vi "S4GUI.vi"(7 "Tab ObsEng":enum32{"Obs", "CCD modes", "Eng"}(tab)) -> ()   [LabVIEW 2018] (continued)
            n3430 = call-dynamic "Read Channel.vi"("error in (no error)"=w7850, "Acquisition in"=w7851) -> ("error out"=w7852:errorcluster, "Channel.lvclass"=w7853:refnum<class "Channel.lvclass">, "Acquisition out"=w7864:refnum<class "Acquisition.lvclass">)  [unwired: 7 in]
            n3431 = call-dynamic "Read Interface.vi"("error in (no error)"=w7852, "Channel in"=w7853) -> ("error out"=w7874:errorcluster, "Interface.lvclass"=w7875:refnum<class "Interface.lvclass">, "Channel out"=w7873:refnum<class "Channel.lvclass">)  [unwired: 7 in]
            n3432 = call "Write Exposure Time.vi"("error in (no error)"=w7874, "Exposure Time"="Exptime ch1", "Interface in"=w7875) -> ("error out"=w7820:errorcluster, "Interface out"=w7821:refnum<class "Interface.lvclass">)  [unwired: 7 in]
            n3433 = case shown="Default" w7807 {
              tunnel: w7821 -> [w7902 w7907]
              tunnel: w7820 -> [w7901 w7906]
              tunnel: "Exptime ch1" -> [_ w7905]
              tunnel: [w7901 w7904] -> w7818
              tunnel: [w7902 w7903] -> w7817
              frame "ZERO" {
              }
              frame Default {
                n3434 = call-dynamic "Write prev ExpTime.vi"("error in (no error)"=w7906, "prev ExpTime"=w7905, "Interface in"=w7907) -> ("error out"=w7904:errorcluster, "Interface out"=w7903:refnum<class "Interface.lvclass">)  [unwired: 7 in]
              }
            }
            n3435 = call-dynamic "Write Suffix.vi"("error in (no error)"=w7818, "Suffix"=w7849, "Interface in"=w7817) -> ("error out"=w7872:errorcluster, "Interface out"=w7871:refnum<class "Interface.lvclass">)  [unwired: 7 in]
            n3436 = call-dynamic "Write ObsType.vi"("error in (no error)"=w7872, "ObsType"=w7847, "Interface in"=w7871) -> ("error out"=w7869:errorcluster, "Interface out"=w7870:refnum<class "Interface.lvclass">)  [unwired: 7 in]
            n3437 = call-dynamic "Write Object.vi"("error in (no error)"=w7869, "Object"=w7846, "Interface in"=w7870) -> ("error out"=w7868:errorcluster, "Interface out"=w7867:refnum<class "Interface.lvclass">)  [unwired: 7 in]
            n3438 = call-dynamic "Write Comments.vi"("error in (no error)"=w7868, "Comments"=w7848, "Interface in"=w7867) -> ("error out"=w7865:errorcluster, "Interface out"=w7866:refnum<class "Interface.lvclass">)  [unwired: 7 in]
            n3439 = call-dynamic "Write DS9.vi"("error in (no error)"=w7865, "DS9"="F", "Interface in"=w7866) -> ("error out"=w7843:errorcluster, "Interface out"=w7845:refnum<class "Interface.lvclass">)  [unwired: 7 in]
            n3440 = call-dynamic "Write Observer.vi"("error in (no error)"=w7843, "Observer"=w7841, "Interface in"=w7845) -> ("error out"=w7842:errorcluster, "Interface out"=w7844:refnum<class "Interface.lvclass">)  [unwired: 7 in]
            n3441 = call-dynamic "Write # Images.vi"("error in (no error)"=w7842, "# Images"="Exp ch1", "Interface in"=w7844) -> ("error out"=w7861:errorcluster, "Interface out"=w7863:refnum<class "Interface.lvclass">)  [unwired: 7 in]
            n3442 = call-dynamic "Write Interface.vi"("error in (no error)"=w7861, "Interface.lvclass"=w7863, "Channel in"=w7873) -> ("error out"=w7854:errorcluster, "Channel out"=w7855:refnum<class "Channel.lvclass">)  [unwired: 7 in]
            n3443 = property on="Exposure Time ch1" class="Slide (strict)"("Scale.Maximum"="Exptime ch1", "Scale.Minimum"=0.0 ("Scale.Range:Minimum")) -> ()  [unwired: 2 in, 2 out]
            n3444 = property on="Cycles Done ch1" class="Slide (strict)"("Scale.Maximum"=w7832, "Scale.Minimum"=0.0 ("Scale.Range:Minimum")) -> ()  [unwired: 2 in, 2 out]
            n3445 = property on="Exposures Done ch1" class="Slide (strict)"("Scale.Maximum"="Exp ch1", "Scale.Minimum"=0.0 ("Scale.Range:Minimum")) -> ()  [unwired: 2 in, 2 out]
            n3446 = call-dynamic "Write ciclos.vi"("error in (no error)"=w7854, "ciclos"=w7832, "Channel in"=w7855) -> ("error out"=w7839:errorcluster, "Channel out"=w7840:refnum<class "Channel.lvclass">)  [unwired: 7 in]
            n3447 = call-dynamic "Write sequencias.vi"("error in (no error)"=w7839, "sequencias"=w7822, "Channel in"=w7840) -> ("error out"=w7838:errorcluster, "Channel out"=w7837:refnum<class "Channel.lvclass">)  [unwired: 7 in]
            n3448 = call-dynamic "Write Channel.vi"("error in (no error)"=w7838, "Channel.lvclass"=w7837, "Acquisition in"=w7864) -> ("error out"=w7805:errorcluster, "Acquisition out"=w7806:refnum<class "Acquisition.lvclass">)  [unwired: 7 in]
            n3449 = call-dynamic "CalcCubeDuration.vi"("error in (no error)"=w7805, "Acquisition in"=w7806) -> ("error out"=w7803:errorcluster, "Acquisition out"=w7804:refnum<class "Acquisition.lvclass">)  [unwired: 8 in]
            n3450 = call-dynamic "Write sequencias.vi"("error in (no error)"=w7803, "sequencias"=w7822, "S4GUI in"=w7813) -> ("error out"=w7834:errorcluster, "S4GUI out"=w7833:refnum<class "S4GUI.lvclass">)  [unwired: 7 in]
            n3451 = call-dynamic "Write ciclos.vi"("error in (no error)"=w7834, "ciclos"=w7832, "S4ACS_GUI in"=w7833) -> ("error out"=w7835:errorcluster, "S4ACS_GUI out"=w7836:refnum<class "S4GUI.lvclass">)  [unwired: 7 in]
            n3452 = call-dynamic "Write TotalCiclos.vi"("error in (no error)"=w7835, "TotalCiclos"=w7832, "S4GUI in"=w7836) -> ("error out"=w7830:errorcluster, "S4GUI out"=w7831:refnum<class "S4GUI.lvclass">)  [unwired: 7 in]
          }
        }
        n3453 = call-dynamic "Write AcquisitionA.vi"("error in (no error)"=w7748, "Acquisition.lvclass"=w7763, "S4ACS_GUI in"=w7764) -> ("error out"=w7749:errorcluster, "S4ACS_GUI out"=w7750:refnum<class "S4GUI.lvclass">)  [unwired: 7 in]
      }
      event "Start ch2": Value Change {
        n3454 = event-data() -> ()  [unwired: 1 in, 6 out]
        n3455 = call "Read Instrument.lvclass.vi"("error in (no error)"=w7916, "S4ACS_GUI in"=w7917) -> ("error out"=w7918:errorcluster, "Instrument.lvclass"=w7919:refnum<class "Instrument.lvclass">, "S4ACS_GUI out"=w7915:refnum<class "S4GUI.lvclass">)  [unwired: 7 in]
        n3456 = call-dynamic "Read mode.vi"("error in (no error)"=w7918, "Instrument in"=w7919) -> ("error out"=w7914:errorcluster, "mode"=w7913:bool)  [unwired: 7 in, 1 out]
        n3457 = call "Read AcquisitionB.vi"("error in (no error)"=w7914, "S4ACS_GUI in"=w7915) -> ("error out"=w7933:errorcluster, "Acquisition.lvclass"=w7934:refnum<class "Acquisition.lvclass">, "S4ACS_GUI out"=w7936:refnum<class "S4GUI.lvclass">)  [unwired: 7 in]
        n3458 = call-dynamic "Read Acq_state.vi"("error in (no error)"=w7933, "Acquisition in"=w7934) -> ("error out"=w7930:errorcluster, "Acq_state"=w7932:u32, "Acquisition out"=w7929:refnum<class "Acquisition.lvclass">)  [unwired: 7 in]
        n3459 = Not Equal?(x=w7932, y=u32 400) -> (x != y?=w7935:bool)
        n3460 = case shown="True" w7935 {
          tunnel: w7936 -> [w7949 w7989]
          tunnel: [w7949 w7996] -> w7928
          tunnel: [w7944 w7995] -> w7912
          tunnel: w7930 -> [w7951 w7976]
          tunnel: w7929 -> [w7954 w7979]
          tunnel: [w7945 w7967] -> w7927
          tunnel: w7925 -> [_ w8017]
          tunnel: w7924 -> [_ w8016]
          tunnel: w7922 -> [_ w8012]
          tunnel: w7921 -> [_ w8011]
          tunnel: w7920 -> [_ w8005]
          tunnel: w7913 -> [_ w7987]
          tunnel: w7911 -> [_ w7974]
          tunnel: w7910 -> [_ w7973]
          tunnel: w7909 -> [_ w7972]
          tunnel: w7908 -> [_ w7971]
          frame False {
            n3461 = call-dynamic "Read Acq_prevstate.vi"("error in (no error)"=w7951, "Acquisition in"=w7954) -> ("error out"=w7950:errorcluster, "Acq_prevstate"=w7952:u32, "Acquisition out"=w7953:refnum<class "Acquisition.lvclass">)  [unwired: 7 in]
            n3462 = call-dynamic "Write Acq_state.vi"("error in (no error)"=w7950, "Acq_state"=w7952, "Acquisition in"=w7953) -> ("error out"=w7941:errorcluster, "Acquisition out"=w7943:refnum<class "Acquisition.lvclass">)  [unwired: 7 in]
            n3463 = call-dynamic "Read enabled.vi"("error in (no error)"=w7941, "Server in"=w7943) -> ("error out"=w7940:errorcluster, "enabled"=w7937:bool, "Server out"=w7942:refnum<class "Acquisition.lvclass">)  [unwired: 7 in]
            n3464 = call-dynamic "Read Channel.vi"("error in (no error)"=w7940, "Acquisition in"=w7942) -> ("error out"=w7938:errorcluster, "Channel.lvclass"=w7939:refnum<class "Channel.lvclass">, "Acquisition out"=w7948:refnum<class "Acquisition.lvclass">)  [unwired: 7 in]
            n3465 = case shown="True" w7937 {
              tunnel: w7939 -> [w7956 w7966]
              tunnel: [w7956 w7964] -> w7947
              tunnel: w7938 -> [w7955 w7961]
              tunnel: [w7955 w7959] -> w7946
              frame False {
              }
              frame True {
                n3466 = call-dynamic "Read State Machine.vi"("error in (no error)"=w7961, "Device in"=w7966) -> ("error out"=w7957:errorcluster, "State Machine.lvclass"=w7958:refnum<class "State Machine.lvclass">, "Device out"=w7965:refnum<class "Channel.lvclass">)  [unwired: 7 in]
                n3467 = call "Next State.vi"("error in (no error)"=w7957, "New_State"=96, "State Machine in"=w7958) -> ("error out"=w7960:errorcluster, "State Machine out"=w7963:refnum<class "State Machine.lvclass">)  [unwired: 7 in]
                n3468 = call-dynamic "Write State Machine.vi"("error in (no error)"=w7960, "State Machine.lvclass"=w7963, "Device in"=w7965) -> ("error out"=w7959:errorcluster, "Device out"=w7964:refnum<class "Channel.lvclass">)  [unwired: 7 in]
              }
            }
            n3469 = call-dynamic "Write Channel.vi"("error in (no error)"=w7946, "Channel.lvclass"=w7947, "Acquisition in"=w7948) -> ("error out"=w7944:errorcluster, "Acquisition out"=w7945:refnum<class "Acquisition.lvclass">)  [unwired: 7 in]
          }
          frame True {
            # "obs type"
            # "suffix"
            # "object"
            n3470 = call "Read Instrument.lvclass.vi"("S4ACS_GUI in"=w7989) -> ("error out"=w7991:errorcluster, "Instrument.lvclass"=w7993:refnum<class "Instrument.lvclass">, "S4ACS_GUI out"=w7980:refnum<class "S4GUI.lvclass">)  [unwired: 8 in]
            n3471 = call "Read WPROT.vi"("error in (no error)"=w7991, "Instrument in"=w7993) -> ("error out"=w7990:errorcluster, "Opt_Selector.lvclass"=w7992:refnum<class "Opt_Selector.lvclass">)  [unwired: 7 in, 1 out]
            n3472 = call-dynamic "Read sequencia.vi"("error in (no error)"=w7990, "Opt_Selector in"=w7992) -> ("sequencia"=w7986:u16)  [unwired: 7 in, 2 out]
            n3473 = case shown="Default" w7974 {
              tunnel: [u32 1 ("#cycles ch2") "#cycles ch2"] -> w7994
              tunnel: [u32 1 w8047] -> w7988
              tunnel: w7987 -> [_ w8046]
              tunnel: w7986 -> [_ w8045]
              frame "FOCUS" {
              }
              frame Default {
                n3474 = case shown="True" w8046 {
                  tunnel: [0 w8051] -> w8047
                  tunnel: w8045 -> [_ w8050]
                  frame False {
                    # "OV 20230424: \n#SEQ agora armazena as\nposições da lâmina utilizadas.\nNa fotometria, #SEQ=0"
                    # "fotometria:"
                  }
                  frame True {
                    # "OV 20230424: \n#SEQ agora armazena as\nposições da lâmina utilizadas.\nNa polarimetria, #SEQ=WPROT.sequencia"
                    # "polarimetria:"
                    n3475 = To Unsigned Long Integer(number=w8050) -> (unsigned 32bit integer=w8051:u32)
                  }
                }
              }
            }
            n3476 = case shown="Default" w7974 {
              tunnel: [u32 271 ("Obs_state") u32 251 ("Obs_state")] -> w7977
              tunnel: w7976 -> [w8055 w8066]
              tunnel: [w8054 w8066] -> w7975
              tunnel: w7973 -> [w8062 _]
              tunnel: w7972 -> [w8061 _]
              tunnel: w7971 -> [w8060 _]
              tunnel: w7980 -> [w8053 w8065]
              tunnel: [w8052 w8065] -> w7978
              frame "FOCUS" {
                n3477 = call-dynamic "Read TelFocus.lvclass.vi"("error in (no error)"=w8055, "S4GUI in"=w8053) -> ("error out"=w8057:errorcluster, "TelFocus.lvclass"=w8059:refnum<class "TelFocus.lvclass">, "S4GUI out"=w8063:refnum<class "S4GUI.lvclass">)  [unwired: 7 in]
                n3478 = call-dynamic "LoadParam.vi"("#steps"=w8060, "error in (no error)"=w8057, "step"=w8061, "init"=w8062, "TelFocus in"=w8059) -> ("error out"=w8056:errorcluster, "TelFocus out"=w8058:refnum<class "TelFocus.lvclass">)  [unwired: 5 in]
                n3479 = call-dynamic "Write TelFocus.lvclass.vi"("error in (no error)"=w8056, "TelFocus.lvclass"=w8058, "S4GUI in"=w8063) -> ("error out"=w8054:errorcluster, "S4GUI out"=w8052:refnum<class "S4GUI.lvclass">)  [unwired: 7 in]
              }
              frame Default {
              }
            }
            n3480 = property on="Start ch2" class="Bool"(error in=w7976, "DisabledEnum"=T12."Disabled and Grayed Out" ("Disabled")) -> ()  [unwired: 1 in, 2 out]
            n3481 = call-dynamic "Write Acq_state.vi"("error in (no error)"=w7975, "Acq_state"=w7977, "Acquisition in"=w7979) -> ("error out"=w8019:errorcluster, "Acquisition out"=w8020:refnum<class "Acquisition.lvclass">)  [unwired: 7 in]
            n3482 = call-dynamic "Read Channel.vi"("error in (no error)"=w8019, "Acquisition in"=w8020) -> ("error out"=w8021:errorcluster, "Channel.lvclass"=w8022:refnum<class "Channel.lvclass">, "Acquisition out"=w8029:refnum<class "Acquisition.lvclass">)  [unwired: 7 in]
            n3483 = call-dynamic "Read Interface.vi"("error in (no error)"=w8021, "Channel in"=w8022) -> ("error out"=w8041:errorcluster, "Interface.lvclass"=w8042:refnum<class "Interface.lvclass">, "Channel out"=w8040:refnum<class "Channel.lvclass">)  [unwired: 7 in]
            n3484 = call "Write Exposure Time.vi"("error in (no error)"=w8041, "Exposure Time"="Exptime ch2", "Interface in"=w8042) -> ("error out"=w7983:errorcluster, "Interface out"=w7985:refnum<class "Interface.lvclass">)  [unwired: 7 in]
            n3485 = case shown="Default" w7974 {
              tunnel: w7985 -> [w8069 w8074]
              tunnel: [w8069 w8073] -> w7984
              tunnel: w7983 -> [w8068 w8072]
              tunnel: [w8068 w8071] -> w7982
              tunnel: "Exptime ch2" -> [_ w8070]
              frame "ZERO" {
              }
              frame Default {
                n3486 = call-dynamic "Write prev ExpTime.vi"("error in (no error)"=w8072, "prev ExpTime"=w8070, "Interface in"=w8074) -> ("error out"=w8071:errorcluster, "Interface out"=w8073:refnum<class "Interface.lvclass">)  [unwired: 7 in]
              }
            }
            n3487 = call-dynamic "Write # Index.vi"("error in (no error)"=w7982, "# Index"="Index ch2", "Interface in"=w7984) -> ("error out"=w8038:errorcluster, "Interface out"=w8039:refnum<class "Interface.lvclass">)  [unwired: 7 in]
            n3488 = call-dynamic "Write Suffix.vi"("error in (no error)"=w8038, "Suffix"=w8017, "Interface in"=w8039) -> ("error out"=w8037:errorcluster, "Interface out"=w8036:refnum<class "Interface.lvclass">)  [unwired: 7 in]
            n3489 = call-dynamic "Write ObsType.vi"("error in (no error)"=w8037, "ObsType"=w8012, "Interface in"=w8036) -> ("error out"=w8034:errorcluster, "Interface out"=w8035:refnum<class "Interface.lvclass">)  [unwired: 7 in]
            n3490 = call-dynamic "Write Object.vi"("error in (no error)"=w8034, "Object"=w8011, "Interface in"=w8035) -> ("error out"=w8033:errorcluster, "Interface out"=w8032:refnum<class "Interface.lvclass">)  [unwired: 7 in]
            n3491 = call-dynamic "Write Comments.vi"("error in (no error)"=w8033, "Comments"=w8016, "Interface in"=w8032) -> ("error out"=w8030:errorcluster, "Interface out"=w8031:refnum<class "Interface.lvclass">)  [unwired: 7 in]
            n3492 = call-dynamic "Write DS9.vi"("error in (no error)"=w8030, "DS9"="F", "Interface in"=w8031) -> ("error out"=w8008:errorcluster, "Interface out"=w8010:refnum<class "Interface.lvclass">)  [unwired: 7 in]
            n3493 = call-dynamic "Write Observer.vi"("error in (no error)"=w8008, "Observer"=w8005, "Interface in"=w8010) -> ("error out"=w8007:errorcluster, "Interface out"=w8009:refnum<class "Interface.lvclass">)  [unwired: 7 in]
            n3494 = call-dynamic "Write # Images.vi"("error in (no error)"=w8007, "# Images"="Exp ch2", "Interface in"=w8009) -> ("error out"=w8014:errorcluster, "Interface out"=w8013:refnum<class "Interface.lvclass">)  [unwired: 7 in]
            n3495 = property on="Exposure Time ch2" class="Slide (strict)"("Scale.Maximum"="Exptime ch2", "Scale.Minimum"=0.0 ("Scale.Range:Minimum")) -> ()  [unwired: 2 in, 2 out]
            n3496 = call-dynamic "Write Interface.vi"("error in (no error)"=w8014, "Interface.lvclass"=w8013, "Channel in"=w8040) -> ("error out"=w8023:errorcluster, "Channel out"=w8024:refnum<class "Channel.lvclass">)  [unwired: 7 in]
            n3497 = property on="Cycles Done ch2" class="Slide (strict)"("Scale.Maximum"=w7994, "Scale.Minimum"=0.0 ("Scale.Range:Minimum")) -> ()  [unwired: 2 in, 2 out]
            n3498 = property on="Exposures Done ch2" class="Slide (strict)"("Scale.Maximum"="Exp ch2", "Scale.Minimum"=0.0 ("Scale.Range:Minimum")) -> ()  [unwired: 2 in, 2 out]
            n3499 = call-dynamic "Write ciclos.vi"("error in (no error)"=w8023, "ciclos"=w7994, "Channel in"=w8024) -> ("error out"=w8004:errorcluster, "Channel out"=w8003:refnum<class "Channel.lvclass">)  [unwired: 7 in]
            n3500 = call-dynamic "Write sequencias.vi"("error in (no error)"=w8004, "sequencias"=w7988, "Channel in"=w8003) -> ("error out"=w8002:errorcluster, "Channel out"=w8001:refnum<class "Channel.lvclass">)  [unwired: 7 in]
            n3501 = call-dynamic "Write Channel.vi"("error in (no error)"=w8002, "Channel.lvclass"=w8001, "Acquisition in"=w8029) -> ("error out"=w7969:errorcluster, "Acquisition out"=w7970:refnum<class "Acquisition.lvclass">)  [unwired: 7 in]
            n3502 = call-dynamic "CalcCubeDuration.vi"("error in (no error)"=w7969, "Acquisition in"=w7970) -> ("error out"=w7968:errorcluster, "Acquisition out"=w7967:refnum<class "Acquisition.lvclass">)  [unwired: 8 in]
            n3503 = call-dynamic "Write sequencias.vi"("error in (no error)"=w7968, "sequencias"=w7988, "S4GUI in"=w7978) -> ("error out"=w7998:errorcluster, "S4GUI out"=w7997:refnum<class "S4GUI.lvclass">)  [unwired: 7 in]
            n3504 = call-dynamic "Write ciclos.vi"("error in (no error)"=w7998, "ciclos"=w7994, "S4ACS_GUI in"=w7997) -> ("error out"=w7999:errorcluster, "S4ACS_GUI out"=w8000:refnum<class "S4GUI.lvclass">)  [unwired: 7 in]
            n3505 = call-dynamic "Write TotalCiclos.vi"("error in (no error)"=w7999, "TotalCiclos"=w7994, "S4GUI in"=w8000) -> ("error out"=w7995:errorcluster, "S4GUI out"=w7996:refnum<class "S4GUI.lvclass">)  [unwired: 7 in]
          }
        }
        n3506 = call "Write AcquisitionB.vi"("error in (no error)"=w7912, "Acquisition.lvclass"=w7927, "S4ACS_GUI in"=w7928) -> ("error out"=w7926:errorcluster, "S4ACS_GUI out"=w7923:refnum<class "S4GUI.lvclass">)  [unwired: 7 in]
      }
      event "Start ch3": Value Change {
        n3507 = event-data() -> ()  [unwired: 1 in, 6 out]
        n3508 = call "Read Instrument.lvclass.vi"("error in (no error)"=w8082, "S4ACS_GUI in"=w8084) -> ("error out"=w8085:errorcluster, "Instrument.lvclass"=w8086:refnum<class "Instrument.lvclass">, "S4ACS_GUI out"=w8083:refnum<class "S4GUI.lvclass">)  [unwired: 7 in]
        n3509 = call-dynamic "Read mode.vi"("error in (no error)"=w8085, "Instrument in"=w8086) -> ("error out"=w8081:errorcluster, "mode"=w8080:bool)  [unwired: 7 in, 1 out]
        n3510 = call-dynamic "Read AcquisitionC.vi"("error in (no error)"=w8081, "S4ACS_GUI in"=w8083) -> ("error out"=w8100:errorcluster, "Acquisition.lvclass"=w8101:refnum<class "Acquisition.lvclass">, "S4ACS_GUI out"=w8103:refnum<class "S4GUI.lvclass">)  [unwired: 7 in]
        n3511 = call-dynamic "Read Acq_state.vi"("error in (no error)"=w8100, "Acquisition in"=w8101) -> ("error out"=w8097:errorcluster, "Acq_state"=w8099:u32, "Acquisition out"=w8096:refnum<class "Acquisition.lvclass">)  [unwired: 7 in]
        n3512 = Not Equal?(x=w8099, y=u32 400) -> (x != y?=w8102:bool)
        n3513 = case shown="True" w8102 {
          tunnel: w8103 -> [w8116 w8153]
          tunnel: [w8116 w8161] -> w8095
          tunnel: [w8111 w8162] -> w8079
          tunnel: w8097 -> [w8118 w8145]
          tunnel: w8096 -> [w8121 w8146]
          tunnel: [w8112 w8134] -> w8094
          tunnel: w8092 -> [_ w8182]
          tunnel: w8091 -> [_ w8181]
          tunnel: w8089 -> [_ w8177]
          tunnel: w8088 -> [_ w8176]
          tunnel: w8087 -> [_ w8171]
          tunnel: w8080 -> [_ w8158]
          tunnel: w8078 -> [_ w8141]
          tunnel: w8077 -> [_ w8140]
          tunnel: w8076 -> [_ w8139]
          tunnel: w8075 -> [_ w8138]
          frame False {
            n3514 = call-dynamic "Read Acq_prevstate.vi"("error in (no error)"=w8118, "Acquisition in"=w8121) -> ("error out"=w8117:errorcluster, "Acq_prevstate"=w8119:u32, "Acquisition out"=w8120:refnum<class "Acquisition.lvclass">)  [unwired: 7 in]
            n3515 = call-dynamic "Write Acq_state.vi"("error in (no error)"=w8117, "Acq_state"=w8119, "Acquisition in"=w8120) -> ("error out"=w8106:errorcluster, "Acquisition out"=w8108:refnum<class "Acquisition.lvclass">)  [unwired: 7 in]
            n3516 = call-dynamic "Read enabled.vi"("error in (no error)"=w8106, "Server in"=w8108) -> ("error out"=w8105:errorcluster, "enabled"=w8104:bool, "Server out"=w8107:refnum<class "Acquisition.lvclass">)  [unwired: 7 in]
            n3517 = call-dynamic "Read Channel.vi"("error in (no error)"=w8105, "Acquisition in"=w8107) -> ("error out"=w8109:errorcluster, "Channel.lvclass"=w8110:refnum<class "Channel.lvclass">, "Acquisition out"=w8114:refnum<class "Acquisition.lvclass">)  [unwired: 7 in]
            n3518 = case shown="True" w8104 {
              tunnel: w8110 -> [w8123 w8133]
              tunnel: [w8123 w8131] -> w8113
              tunnel: w8109 -> [w8122 w8128]
              tunnel: [w8122 w8126] -> w8115
              frame False {
              }
              frame True {
                n3519 = call-dynamic "Read State Machine.vi"("error in (no error)"=w8128, "Device in"=w8133) -> ("error out"=w8124:errorcluster, "State Machine.lvclass"=w8125:refnum<class "State Machine.lvclass">, "Device out"=w8132:refnum<class "Channel.lvclass">)  [unwired: 7 in]
                n3520 = call "Next State.vi"("error in (no error)"=w8124, "New_State"=96, "State Machine in"=w8125) -> ("error out"=w8127:errorcluster, "State Machine out"=w8130:refnum<class "State Machine.lvclass">)  [unwired: 7 in]
                n3521 = call-dynamic "Write State Machine.vi"("error in (no error)"=w8127, "State Machine.lvclass"=w8130, "Device in"=w8132) -> ("error out"=w8126:errorcluster, "Device out"=w8131:refnum<class "Channel.lvclass">)  [unwired: 7 in]
              }
            }
            n3522 = call-dynamic "Write Channel.vi"("error in (no error)"=w8115, "Channel.lvclass"=w8113, "Acquisition in"=w8114) -> ("error out"=w8111:errorcluster, "Acquisition out"=w8112:refnum<class "Acquisition.lvclass">)  [unwired: 7 in]
          }
          frame True {
            # "obs type"
            # "suffix"
            # "object"
            n3523 = call "Read Instrument.lvclass.vi"("S4ACS_GUI in"=w8153) -> ("error out"=w8155:errorcluster, "Instrument.lvclass"=w8157:refnum<class "Instrument.lvclass">, "S4ACS_GUI out"=w8144:refnum<class "S4GUI.lvclass">)  [unwired: 8 in]
            n3524 = call "Read WPROT.vi"("error in (no error)"=w8155, "Instrument in"=w8157) -> ("error out"=w8154:errorcluster, "Opt_Selector.lvclass"=w8156:refnum<class "Opt_Selector.lvclass">)  [unwired: 7 in, 1 out]
            n3525 = call-dynamic "Read sequencia.vi"("error in (no error)"=w8154, "Opt_Selector in"=w8156) -> ("sequencia"=w8152:u16)  [unwired: 7 in, 2 out]
            n3526 = case shown="\"FOCUS\"" w8141 {
              tunnel: [u32 271 ("Obs_state") u32 251 ("Obs_state")] -> w8142
              tunnel: w8145 -> [w8221 w8232]
              tunnel: [w8220 w8232] -> _
              tunnel: w8140 -> [w8228 _]
              tunnel: w8139 -> [w8227 _]
              tunnel: w8138 -> [w8226 _]
              tunnel: w8144 -> [w8219 w8231]
              tunnel: [w8218 w8231] -> w8143
              frame "FOCUS" {
                n3527 = call-dynamic "Read TelFocus.lvclass.vi"("error in (no error)"=w8221, "S4GUI in"=w8219) -> ("error out"=w8223:errorcluster, "TelFocus.lvclass"=w8225:refnum<class "TelFocus.lvclass">, "S4GUI out"=w8229:refnum<class "S4GUI.lvclass">)  [unwired: 7 in]
                n3528 = call-dynamic "LoadParam.vi"("#steps"=w8226, "error in (no error)"=w8223, "step"=w8227, "init"=w8228, "TelFocus in"=w8225) -> ("error out"=w8222:errorcluster, "TelFocus out"=w8224:refnum<class "TelFocus.lvclass">)  [unwired: 5 in]
                n3529 = call-dynamic "Write TelFocus.lvclass.vi"("error in (no error)"=w8222, "TelFocus.lvclass"=w8224, "S4GUI in"=w8229) -> ("error out"=w8220:errorcluster, "S4GUI out"=w8218:refnum<class "S4GUI.lvclass">)  [unwired: 7 in]
              }
              frame Default {
              }
            }
            n3530 = case shown="Default" w8141 {
              tunnel: [u32 1 ("#cycles ch3") "#cycles ch3"] -> w8160
              tunnel: [u32 1 w8213] -> w8159
              tunnel: w8158 -> [_ w8212]
              tunnel: w8152 -> [_ w8211]
              frame "FOCUS" {
                # "PARA A SEQUÊNCIA DE FOCO, #CYCLES=1 E #SEQS=1"
              }
              frame Default {
                n3531 = case shown="True" w8212 {
                  tunnel: [0 w8217] -> w8213
                  tunnel: w8211 -> [_ w8216]
                  frame False {
                    # "OV 20230424: \n#SEQ agora armazena as\nposições da lâmina utilizadas.\nNa fotometria, #SEQ=0"
                    # "fotometria:"
                  }
                  frame True {
                    # "OV 20230424: \n#SEQ agora armazena as\nposições da lâmina utilizadas.\nNa polarimetria, #SEQ=WPROT.sequencia"
                    # "polarimetria:"
                    n3532 = To Unsigned Long Integer(number=w8216) -> (unsigned 32bit integer=w8217:u32)
                  }
                }
              }
            }
            n3533 = call-dynamic "Write Acq_state.vi"("Acq_state"=w8142, "Acquisition in"=w8146) -> ("error out"=w8184:errorcluster, "Acquisition out"=w8185:refnum<class "Acquisition.lvclass">)  [unwired: 8 in]
            n3534 = call-dynamic "Read Channel.vi"("error in (no error)"=w8184, "Acquisition in"=w8185) -> ("error out"=w8186:errorcluster, "Channel.lvclass"=w8187:refnum<class "Channel.lvclass">, "Acquisition out"=w8195:refnum<class "Acquisition.lvclass">)  [unwired: 7 in]
            n3535 = property on="Start ch3" class="Bool"(error in=w8145, "DisabledEnum"=T12."Disabled and Grayed Out" ("Disabled")) -> ()  [unwired: 1 in, 2 out]
            n3536 = call-dynamic "Read Interface.vi"("error in (no error)"=w8186, "Channel in"=w8187) -> ("error out"=w8207:errorcluster, "Interface.lvclass"=w8208:refnum<class "Interface.lvclass">, "Channel out"=w8206:refnum<class "Channel.lvclass">)  [unwired: 7 in]
            n3537 = call "Write Exposure Time.vi"("error in (no error)"=w8207, "Exposure Time"="Exptime ch3", "Interface in"=w8208) -> ("error out"=w8149:errorcluster, "Interface out"=w8150:refnum<class "Interface.lvclass">)  [unwired: 7 in]
            n3538 = case shown="\"ZERO\"" w8141 {
              tunnel: [w8234 w8240] -> w8151
              tunnel: w8150 -> [w8234 w8239]
              tunnel: w8149 -> [w8235 w8238]
              tunnel: [w8235 w8237] -> w8148
              tunnel: "Exptime ch3" -> [_ w8236]
              frame "ZERO" {
              }
              frame Default {
                n3539 = call-dynamic "Write prev ExpTime.vi"("error in (no error)"=w8238, "prev ExpTime"=w8236, "Interface in"=w8239) -> ("error out"=w8237:errorcluster, "Interface out"=w8240:refnum<class "Interface.lvclass">)  [unwired: 7 in]
              }
            }
            n3540 = call-dynamic "Write # Index.vi"("error in (no error)"=w8148, "# Index"="Index ch3", "Interface in"=w8151) -> ("error out"=w8204:errorcluster, "Interface out"=w8205:refnum<class "Interface.lvclass">)  [unwired: 7 in]
            n3541 = call-dynamic "Write Suffix.vi"("error in (no error)"=w8204, "Suffix"=w8182, "Interface in"=w8205) -> ("error out"=w8203:errorcluster, "Interface out"=w8202:refnum<class "Interface.lvclass">)  [unwired: 7 in]
            n3542 = call-dynamic "Write ObsType.vi"("error in (no error)"=w8203, "ObsType"=w8176, "Interface in"=w8202) -> ("error out"=w8200:errorcluster, "Interface out"=w8201:refnum<class "Interface.lvclass">)  [unwired: 7 in]
            n3543 = call-dynamic "Write Object.vi"("error in (no error)"=w8200, "Object"=w8177, "Interface in"=w8201) -> ("error out"=w8199:errorcluster, "Interface out"=w8198:refnum<class "Interface.lvclass">)  [unwired: 7 in]
            n3544 = call-dynamic "Write Comments.vi"("error in (no error)"=w8199, "Comments"=w8181, "Interface in"=w8198) -> ("error out"=w8196:errorcluster, "Interface out"=w8197:refnum<class "Interface.lvclass">)  [unwired: 7 in]
            n3545 = call-dynamic "Write DS9.vi"("error in (no error)"=w8196, "DS9"="F", "Interface in"=w8197) -> ("error out"=w8173:errorcluster, "Interface out"=w8175:refnum<class "Interface.lvclass">)  [unwired: 7 in]
            n3546 = call-dynamic "Write Observer.vi"("error in (no error)"=w8173, "Observer"=w8171, "Interface in"=w8175) -> ("error out"=w8172:errorcluster, "Interface out"=w8174:refnum<class "Interface.lvclass">)  [unwired: 7 in]
            n3547 = call-dynamic "Write # Images.vi"("error in (no error)"=w8172, "# Images"="Exp ch3", "Interface in"=w8174) -> ("error out"=w8178:errorcluster, "Interface out"=w8179:refnum<class "Interface.lvclass">)  [unwired: 7 in]
            n3548 = call-dynamic "Write Interface.vi"("error in (no error)"=w8178, "Interface.lvclass"=w8179, "Channel in"=w8206) -> ("error out"=w8188:errorcluster, "Channel out"=w8189:refnum<class "Channel.lvclass">)  [unwired: 7 in]
            n3549 = property on="Exposure Time ch3" class="Slide (strict)"("Scale.Maximum"="Exptime ch3", "Scale.Minimum"=0.0 ("Scale.Range:Minimum")) -> ()  [unwired: 2 in, 2 out]
            n3550 = property on="Exposures Done ch3" class="Slide (strict)"("Scale.Maximum"="Exp ch3", "Scale.Minimum"=0.0 ("Scale.Range:Minimum")) -> ()  [unwired: 2 in, 2 out]
            n3551 = property on="Cycles Done ch3" class="Slide (strict)"("Scale.Maximum"=w8160, "Scale.Minimum"=0.0 ("Scale.Range:Minimum")) -> ()  [unwired: 2 in, 2 out]
            n3552 = call-dynamic "Write ciclos.vi"("error in (no error)"=w8188, "ciclos"=w8160, "Channel in"=w8189) -> ("error out"=w8169:errorcluster, "Channel out"=w8170:refnum<class "Channel.lvclass">)  [unwired: 7 in]
            n3553 = call-dynamic "Write sequencias.vi"("error in (no error)"=w8169, "sequencias"=w8159, "Channel in"=w8170) -> ("error out"=w8167:errorcluster, "Channel out"=w8168:refnum<class "Channel.lvclass">)  [unwired: 7 in]
            n3554 = call-dynamic "Write Channel.vi"("error in (no error)"=w8167, "Channel.lvclass"=w8168, "Acquisition in"=w8195) -> ("error out"=w8136:errorcluster, "Acquisition out"=w8137:refnum<class "Acquisition.lvclass">)  [unwired: 7 in]
            n3555 = call-dynamic "CalcCubeDuration.vi"("error in (no error)"=w8136, "Acquisition in"=w8137) -> ("error out"=w8135:errorcluster, "Acquisition out"=w8134:refnum<class "Acquisition.lvclass">)  [unwired: 8 in]
            n3556 = call-dynamic "Write sequencias.vi"("error in (no error)"=w8135, "sequencias"=w8159, "S4GUI in"=w8143) -> ("error out"=w8164:errorcluster, "S4GUI out"=w8163:refnum<class "S4GUI.lvclass">)  [unwired: 7 in]
            n3557 = call-dynamic "Write ciclos.vi"("error in (no error)"=w8164, "ciclos"=w8160, "S4ACS_GUI in"=w8163) -> ("error out"=w8165:errorcluster, "S4ACS_GUI out"=w8166:refnum<class "S4GUI.lvclass">)  [unwired: 7 in]
            n3558 = call-dynamic "Write TotalCiclos.vi"("error in (no error)"=w8165, "TotalCiclos"=w8160, "S4GUI in"=w8166) -> ("error out"=w8162:errorcluster, "S4GUI out"=w8161:refnum<class "S4GUI.lvclass">)  [unwired: 7 in]
          }
        }
        n3559 = call-dynamic "Write AcquisitionC.vi"("error in (no error)"=w8079, "Acquisition.lvclass"=w8094, "S4ACS_GUI in"=w8095) -> ("error out"=w8093:errorcluster, "S4ACS_GUI out"=w8090:refnum<class "S4GUI.lvclass">)  [unwired: 7 in]
      }
      event "Start ch4": Value Change {
        n3560 = event-data() -> ()  [unwired: 1 in, 6 out]
        n3561 = call "Read Instrument.lvclass.vi"("error in (no error)"=w8250, "S4ACS_GUI in"=w8251) -> ("error out"=w8252:errorcluster, "Instrument.lvclass"=w8253:refnum<class "Instrument.lvclass">, "S4ACS_GUI out"=w8249:refnum<class "S4GUI.lvclass">)  [unwired: 7 in]
        n3562 = call-dynamic "Read mode.vi"("error in (no error)"=w8252, "Instrument in"=w8253) -> ("error out"=w8248:errorcluster, "mode"=w8247:bool)  [unwired: 7 in, 1 out]
        n3563 = call-dynamic "Read AcquisitionD.vi"("error in (no error)"=w8248, "S4ACS_GUI in"=w8249) -> ("error out"=w8266:errorcluster, "Acquisition.lvclass"=w8267:refnum<class "Acquisition.lvclass">, "S4ACS_GUI out"=w8269:refnum<class "S4GUI.lvclass">)  [unwired: 7 in]
        n3564 = call-dynamic "Read Acq_state.vi"("error in (no error)"=w8266, "Acquisition in"=w8267) -> ("error out"=w8263:errorcluster, "Acq_state"=w8265:u32, "Acquisition out"=w8262:refnum<class "Acquisition.lvclass">)  [unwired: 7 in]
        n3565 = Not Equal?(x=w8265, y=u32 400) -> (x != y?=w8268:bool)
        n3566 = case shown="False" w8268 {
          tunnel: w8269 -> [w8282 w8320]
          tunnel: [w8278 w8328] -> w8246
          tunnel: w8263 -> [w8284 w8311]
          tunnel: w8262 -> [w8287 w8312]
          tunnel: [w8277 w8300] -> w8261
          tunnel: w8259 -> [_ w8349]
          tunnel: w8258 -> [_ w8348]
          tunnel: w8256 -> [_ w8344]
          tunnel: w8255 -> [_ w8343]
          tunnel: w8254 -> [_ w8338]
          tunnel: w8247 -> [_ w8326]
          tunnel: [w8282 w8329] -> w8245
          tunnel: w8244 -> [_ w8307]
          tunnel: w8243 -> [_ w8306]
          tunnel: w8242 -> [_ w8305]
          tunnel: w8241 -> [_ w8304]
          frame False {
            n3567 = call-dynamic "Read Acq_prevstate.vi"("error in (no error)"=w8284, "Acquisition in"=w8287) -> ("error out"=w8283:errorcluster, "Acq_prevstate"=w8285:u32, "Acquisition out"=w8286:refnum<class "Acquisition.lvclass">)  [unwired: 7 in]
            n3568 = call-dynamic "Write Acq_state.vi"("error in (no error)"=w8283, "Acq_state"=w8285, "Acquisition in"=w8286) -> ("error out"=w8272:errorcluster, "Acquisition out"=w8276:refnum<class "Acquisition.lvclass">)  [unwired: 7 in]
            n3569 = call-dynamic "Read enabled.vi"("error in (no error)"=w8272, "Server in"=w8276) -> ("error out"=w8271:errorcluster, "enabled"=w8270:bool, "Server out"=w8275:refnum<class "Acquisition.lvclass">)  [unwired: 7 in]
            n3570 = call-dynamic "Read Channel.vi"("error in (no error)"=w8271, "Acquisition in"=w8275) -> ("error out"=w8273:errorcluster, "Channel.lvclass"=w8274:refnum<class "Channel.lvclass">, "Acquisition out"=w8280:refnum<class "Acquisition.lvclass">)  [unwired: 7 in]
            n3571 = case shown="True" w8270 {
              tunnel: w8274 -> [w8289 w8299]
              tunnel: [w8289 w8297] -> w8279
              tunnel: w8273 -> [w8288 w8294]
              tunnel: [w8288 w8292] -> w8281
              frame False {
              }
              frame True {
                n3572 = call-dynamic "Read State Machine.vi"("error in (no error)"=w8294, "Device in"=w8299) -> ("error out"=w8290:errorcluster, "State Machine.lvclass"=w8291:refnum<class "State Machine.lvclass">, "Device out"=w8298:refnum<class "Channel.lvclass">)  [unwired: 7 in]
                n3573 = call "Next State.vi"("error in (no error)"=w8290, "New_State"=96, "State Machine in"=w8291) -> ("error out"=w8293:errorcluster, "State Machine out"=w8296:refnum<class "State Machine.lvclass">)  [unwired: 7 in]
                n3574 = call-dynamic "Write State Machine.vi"("error in (no error)"=w8293, "State Machine.lvclass"=w8296, "Device in"=w8298) -> ("error out"=w8292:errorcluster, "Device out"=w8297:refnum<class "Channel.lvclass">)  [unwired: 7 in]
              }
            }
            n3575 = call-dynamic "Write Channel.vi"("error in (no error)"=w8281, "Channel.lvclass"=w8279, "Acquisition in"=w8280) -> ("error out"=w8278:errorcluster, "Acquisition out"=w8277:refnum<class "Acquisition.lvclass">)  [unwired: 7 in]
          }
          frame True {
            # "obs type"
            # "suffix"
            # "object"
            n3576 = call "Read Instrument.lvclass.vi"("S4ACS_GUI in"=w8320) -> ("error out"=w8322:errorcluster, "Instrument.lvclass"=w8324:refnum<class "Instrument.lvclass">, "S4ACS_GUI out"=w8309:refnum<class "S4GUI.lvclass">)  [unwired: 8 in]
            n3577 = call "Read WPROT.vi"("error in (no error)"=w8322, "Instrument in"=w8324) -> ("error out"=w8321:errorcluster, "Opt_Selector.lvclass"=w8323:refnum<class "Opt_Selector.lvclass">)  [unwired: 7 in, 1 out]
            n3578 = call-dynamic "Read sequencia.vi"("error in (no error)"=w8321, "Opt_Selector in"=w8323) -> ("sequencia"=w8319:u16)  [unwired: 7 in, 2 out]
            n3579 = case shown="\"FOCUS\"" w8307 {
              tunnel: [u32 271 ("Obs_state") u32 251 ("Obs_state")] -> w8313
              tunnel: w8311 -> [w8388 w8399]
              tunnel: [w8387 w8399] -> w8310
              tunnel: w8306 -> [w8395 _]
              tunnel: w8305 -> [w8394 _]
              tunnel: w8304 -> [w8393 _]
              tunnel: w8309 -> [w8386 w8398]
              tunnel: [w8385 w8398] -> w8308
              frame "FOCUS" {
                n3580 = call-dynamic "Read TelFocus.lvclass.vi"("error in (no error)"=w8388, "S4GUI in"=w8386) -> ("error out"=w8390:errorcluster, "TelFocus.lvclass"=w8392:refnum<class "TelFocus.lvclass">, "S4GUI out"=w8396:refnum<class "S4GUI.lvclass">)  [unwired: 7 in]
                n3581 = call-dynamic "LoadParam.vi"("#steps"=w8393, "error in (no error)"=w8390, "step"=w8394, "init"=w8395, "TelFocus in"=w8392) -> ("error out"=w8389:errorcluster, "TelFocus out"=w8391:refnum<class "TelFocus.lvclass">)  [unwired: 5 in]
                n3582 = call-dynamic "Write TelFocus.lvclass.vi"("error in (no error)"=w8389, "TelFocus.lvclass"=w8391, "S4GUI in"=w8396) -> ("error out"=w8387:errorcluster, "S4GUI out"=w8385:refnum<class "S4GUI.lvclass">)  [unwired: 7 in]
              }
              frame Default {
              }
            }
            n3583 = case shown="\"FOCUS\"" w8307 {
              tunnel: [u32 1 ("#cycles ch4") "#cycles ch4"] -> w8327
              tunnel: w8326 -> [_ w8380]
              tunnel: [u32 1 w8379] -> w8325
              tunnel: w8319 -> [_ w8378]
              frame "FOCUS" {
                # "Na sequência de foco, #cycles=1 e #seqs=1"
              }
              frame Default {
                n3584 = case shown="True" w8380 {
                  tunnel: [0 w8384] -> w8379
                  tunnel: w8378 -> [_ w8383]
                  frame False {
                    # "OV 20230424: \n#SEQ agora armazena as\nposições da lâmina utilizadas.\nNa fotometria, #SEQ=0"
                    # "fotometria:"
                  }
                  frame True {
                    # "OV 20230424: \n#SEQ agora armazena as\nposições da lâmina utilizadas.\nNa polarimetria, #SEQ=WPROT.sequencia"
                    # "polarimetria:"
                    n3585 = To Unsigned Long Integer(number=w8383) -> (unsigned 32bit integer=w8384:u32)
                  }
                }
              }
            }
            n3586 = call-dynamic "Write Acq_state.vi"("error in (no error)"=w8310, "Acq_state"=w8313, "Acquisition in"=w8312) -> ("error out"=w8351:errorcluster, "Acquisition out"=w8352:refnum<class "Acquisition.lvclass">)  [unwired: 7 in]
            n3587 = call-dynamic "Read Channel.vi"("error in (no error)"=w8351, "Acquisition in"=w8352) -> ("error out"=w8353:errorcluster, "Channel.lvclass"=w8354:refnum<class "Channel.lvclass">, "Acquisition out"=w8362:refnum<class "Acquisition.lvclass">)  [unwired: 7 in]
            n3588 = call-dynamic "Read Interface.vi"("error in (no error)"=w8353, "Channel in"=w8354) -> ("error out"=w8374:errorcluster, "Interface.lvclass"=w8375:refnum<class "Interface.lvclass">, "Channel out"=w8373:refnum<class "Channel.lvclass">)  [unwired: 7 in]
            n3589 = property on="Start ch4" class="Bool"(error in=w8311, "DisabledEnum"=T12."Disabled and Grayed Out" ("Disabled")) -> ()  [unwired: 1 in, 2 out]
            n3590 = call "Write Exposure Time.vi"("error in (no error)"=w8374, "Exposure Time"="Exptime ch4", "Interface in"=w8375) -> ("error out"=w8315:errorcluster, "Interface out"=w8318:refnum<class "Interface.lvclass">)  [unwired: 7 in]
            n3591 = case shown="\"ZERO\"" w8307 {
              tunnel: w8318 -> [w8402 w8407]
              tunnel: [w8402 w8406] -> w8317
              tunnel: [w8401 w8405] -> w8316
              tunnel: w8315 -> [w8401 w8404]
              tunnel: "Exptime ch4" -> [_ w8403]
              frame "ZERO" {
              }
              frame Default {
                n3592 = call-dynamic "Write prev ExpTime.vi"("error in (no error)"=w8404, "prev ExpTime"=w8403, "Interface in"=w8407) -> ("error out"=w8405:errorcluster, "Interface out"=w8406:refnum<class "Interface.lvclass">)  [unwired: 7 in]
              }
            }
            n3593 = call-dynamic "Write # Index.vi"("error in (no error)"=w8316, "# Index"="Index ch4", "Interface in"=w8317) -> ("error out"=w8371:errorcluster, "Interface out"=w8372:refnum<class "Interface.lvclass">)  [unwired: 7 in]
            n3594 = call-dynamic "Write Suffix.vi"("error in (no error)"=w8371, "Suffix"=w8349, "Interface in"=w8372) -> ("error out"=w8370:errorcluster, "Interface out"=w8369:refnum<class "Interface.lvclass">)  [unwired: 7 in]
            n3595 = call-dynamic "Write ObsType.vi"("error in (no error)"=w8370, "ObsType"=w8344, "Interface in"=w8369) -> ("error out"=w8367:errorcluster, "Interface out"=w8368:refnum<class "Interface.lvclass">)  [unwired: 7 in]
            n3596 = call-dynamic "Write Object.vi"("error in (no error)"=w8367, "Object"=w8343, "Interface in"=w8368) -> ("error out"=w8366:errorcluster, "Interface out"=w8365:refnum<class "Interface.lvclass">)  [unwired: 7 in]
            n3597 = call-dynamic "Write Comments.vi"("error in (no error)"=w8366, "Comments"=w8348, "Interface in"=w8365) -> ("error out"=w8363:errorcluster, "Interface out"=w8364:refnum<class "Interface.lvclass">)  [unwired: 7 in]
            n3598 = call-dynamic "Write DS9.vi"("error in (no error)"=w8363, "DS9"="F", "Interface in"=w8364) -> ("error out"=w8340:errorcluster, "Interface out"=w8342:refnum<class "Interface.lvclass">)  [unwired: 7 in]
            n3599 = call-dynamic "Write Observer.vi"("error in (no error)"=w8340, "Observer"=w8338, "Interface in"=w8342) -> ("error out"=w8339:errorcluster, "Interface out"=w8341:refnum<class "Interface.lvclass">)  [unwired: 7 in]
            n3600 = call-dynamic "Write # Images.vi"("error in (no error)"=w8339, "# Images"="Exp ch4", "Interface in"=w8341) -> ("error out"=w8345:errorcluster, "Interface out"=w8346:refnum<class "Interface.lvclass">)  [unwired: 7 in]
            n3601 = property on="Exposure Time ch4" class="Slide (strict)"("Scale.Maximum"="Exptime ch4", "Scale.Minimum"=0.0 ("Scale.Range:Minimum")) -> ()  [unwired: 2 in, 2 out]
            n3602 = property on="Exposures Done ch4" class="Slide (strict)"("Scale.Maximum"="Exp ch4", "Scale.Minimum"=0.0 ("Scale.Range:Minimum")) -> ()  [unwired: 2 in, 2 out]
            n3603 = call-dynamic "Write Interface.vi"("error in (no error)"=w8345, "Interface.lvclass"=w8346, "Channel in"=w8373) -> ("error out"=w8355:errorcluster, "Channel out"=w8356:refnum<class "Channel.lvclass">)  [unwired: 7 in]
            n3604 = property on="Cycles Done ch4" class="Slide (strict)"("Scale.Maximum"=w8327, "Scale.Minimum"=0.0 ("Scale.Range:Minimum")) -> ()  [unwired: 2 in, 2 out]
            n3605 = call-dynamic "Write ciclos.vi"("error in (no error)"=w8355, "ciclos"=w8327, "Channel in"=w8356) -> ("error out"=w8336:errorcluster, "Channel out"=w8337:refnum<class "Channel.lvclass">)  [unwired: 7 in]
            n3606 = call-dynamic "Write sequencias.vi"("error in (no error)"=w8336, "sequencias"=w8325, "Channel in"=w8337) -> ("error out"=w8335:errorcluster, "Channel out"=w8334:refnum<class "Channel.lvclass">)  [unwired: 7 in]
            n3607 = call-dynamic "Write Channel.vi"("error in (no error)"=w8335, "Channel.lvclass"=w8334, "Acquisition in"=w8362) -> ("error out"=w8302:errorcluster, "Acquisition out"=w8303:refnum<class "Acquisition.lvclass">)  [unwired: 7 in]
            n3608 = call-dynamic "CalcCubeDuration.vi"("error in (no error)"=w8302, "Acquisition in"=w8303) -> ("error out"=w8301:errorcluster, "Acquisition out"=w8300:refnum<class "Acquisition.lvclass">)  [unwired: 8 in]
            n3609 = call-dynamic "Write sequencias.vi"("error in (no error)"=w8301, "sequencias"=w8325, "S4GUI in"=w8308) -> ("error out"=w8331:errorcluster, "S4GUI out"=w8330:refnum<class "S4GUI.lvclass">)  [unwired: 7 in]
            n3610 = call-dynamic "Write ciclos.vi"("error in (no error)"=w8331, "ciclos"=w8327, "S4ACS_GUI in"=w8330) -> ("error out"=w8332:errorcluster, "S4ACS_GUI out"=w8333:refnum<class "S4GUI.lvclass">)  [unwired: 7 in]
            n3611 = call-dynamic "Write TotalCiclos.vi"("error in (no error)"=w8332, "TotalCiclos"=w8327, "S4GUI in"=w8333) -> ("error out"=w8328:errorcluster, "S4GUI out"=w8329:refnum<class "S4GUI.lvclass">)  [unwired: 7 in]
          }
        }
        n3612 = call-dynamic "Write AcquisitionD.vi"("error in (no error)"=w8246, "Acquisition.lvclass"=w8261, "S4ACS_GUI in"=w8245) -> ("error out"=w8260:errorcluster, "S4ACS_GUI out"=w8257:refnum<class "S4GUI.lvclass">)  [unwired: 7 in]
      }
      event "Exptime ch1": Value Change {
        n3613 = event-data() -> ("NewVal"=w8412:dbl)  [unwired: 1 in]
        n3614 = call-dynamic "Read AcquisitionA.vi"("error in (no error)"=w8411, "S4ACS_GUI in"=w8410) -> ("error out"=w8426:errorcluster, "Acquisition.lvclass"=w8427:refnum<class "Acquisition.lvclass">, "S4ACS_GUI out"=w8424:refnum<class "S4GUI.lvclass">)  [unwired: 7 in]
        n3615 = call-dynamic "Read Channel.vi"("error in (no error)"=w8426, "Acquisition in"=w8427) -> ("error out"=w8415:errorcluster, "Channel.lvclass"=w8416:refnum<class "Channel.lvclass">, "Acquisition out"=w8417:refnum<class "Acquisition.lvclass">)  [unwired: 7 in]
        n3616 = call-dynamic "Read Interface.vi"("error in (no error)"=w8415, "Channel in"=w8416) -> ("error out"=w8421:errorcluster, "Interface.lvclass"=w8422:refnum<class "Interface.lvclass">, "Channel out"=w8420:refnum<class "Channel.lvclass">)  [unwired: 7 in]
        n3617 = call "Write Exposure Time.vi"("error in (no error)"=w8421, "Exposure Time"=w8412, "Interface in"=w8422) -> ("error out"=w8413:errorcluster, "Interface out"=w8414:refnum<class "Interface.lvclass">)  [unwired: 7 in]
        n3618 = call-dynamic "Write Interface.vi"("error in (no error)"=w8413, "Interface.lvclass"=w8414, "Channel in"=w8420) -> ("error out"=w8419:errorcluster, "Channel out"=w8418:refnum<class "Channel.lvclass">)  [unwired: 7 in]
        n3619 = call-dynamic "Write Channel.vi"("error in (no error)"=w8419, "Channel.lvclass"=w8418, "Acquisition in"=w8417) -> ("error out"=w8423:errorcluster, "Acquisition out"=w8425:refnum<class "Acquisition.lvclass">)  [unwired: 7 in]
        n3620 = call-dynamic "Write AcquisitionA.vi"("error in (no error)"=w8423, "Acquisition.lvclass"=w8425, "S4ACS_GUI in"=w8424) -> ("error out"=w8409:errorcluster, "S4ACS_GUI out"=w8408:refnum<class "S4GUI.lvclass">)  [unwired: 7 in]
      }
      event "Exptime ch2": Value Change {
        n3621 = event-data() -> ("NewVal"=w8432:dbl)  [unwired: 1 in]
        n3622 = call "Read AcquisitionB.vi"("error in (no error)"=w8431, "S4ACS_GUI in"=w8430) -> ("error out"=w8446:errorcluster, "Acquisition.lvclass"=w8447:refnum<class "Acquisition.lvclass">, "S4ACS_GUI out"=w8444:refnum<class "S4GUI.lvclass">)  [unwired: 7 in]
        n3623 = call-dynamic "Read Channel.vi"("error in (no error)"=w8446, "Acquisition in"=w8447) -> ("error out"=w8435:errorcluster, "Channel.lvclass"=w8436:refnum<class "Channel.lvclass">, "Acquisition out"=w8437:refnum<class "Acquisition.lvclass">)  [unwired: 7 in]
        n3624 = call-dynamic "Read Interface.vi"("error in (no error)"=w8435, "Channel in"=w8436) -> ("error out"=w8441:errorcluster, "Interface.lvclass"=w8442:refnum<class "Interface.lvclass">, "Channel out"=w8440:refnum<class "Channel.lvclass">)  [unwired: 7 in]
        n3625 = call "Write Exposure Time.vi"("error in (no error)"=w8441, "Exposure Time"=w8432, "Interface in"=w8442) -> ("error out"=w8433:errorcluster, "Interface out"=w8434:refnum<class "Interface.lvclass">)  [unwired: 7 in]
        n3626 = call-dynamic "Write Interface.vi"("error in (no error)"=w8433, "Interface.lvclass"=w8434, "Channel in"=w8440) -> ("error out"=w8439:errorcluster, "Channel out"=w8438:refnum<class "Channel.lvclass">)  [unwired: 7 in]
        n3627 = call-dynamic "Write Channel.vi"("error in (no error)"=w8439, "Channel.lvclass"=w8438, "Acquisition in"=w8437) -> ("error out"=w8443:errorcluster, "Acquisition out"=w8445:refnum<class "Acquisition.lvclass">)  [unwired: 7 in]
        n3628 = call "Write AcquisitionB.vi"("error in (no error)"=w8443, "Acquisition.lvclass"=w8445, "S4ACS_GUI in"=w8444) -> ("error out"=w8429:errorcluster, "S4ACS_GUI out"=w8428:refnum<class "S4GUI.lvclass">)  [unwired: 7 in]
      }
      event "Exptime ch3": Value Change {
        n3629 = event-data() -> ("NewVal"=w8452:dbl)  [unwired: 1 in]
        n3630 = call-dynamic "Read AcquisitionC.vi"("error in (no error)"=w8451, "S4ACS_GUI in"=w8450) -> ("error out"=w8466:errorcluster, "Acquisition.lvclass"=w8467:refnum<class "Acquisition.lvclass">, "S4ACS_GUI out"=w8464:refnum<class "S4GUI.lvclass">)  [unwired: 7 in]
        n3631 = call-dynamic "Read Channel.vi"("error in (no error)"=w8466, "Acquisition in"=w8467) -> ("error out"=w8455:errorcluster, "Channel.lvclass"=w8456:refnum<class "Channel.lvclass">, "Acquisition out"=w8457:refnum<class "Acquisition.lvclass">)  [unwired: 7 in]
        n3632 = call-dynamic "Read Interface.vi"("error in (no error)"=w8455, "Channel in"=w8456) -> ("error out"=w8461:errorcluster, "Interface.lvclass"=w8462:refnum<class "Interface.lvclass">, "Channel out"=w8460:refnum<class "Channel.lvclass">)  [unwired: 7 in]
        n3633 = call "Write Exposure Time.vi"("error in (no error)"=w8461, "Exposure Time"=w8452, "Interface in"=w8462) -> ("error out"=w8453:errorcluster, "Interface out"=w8454:refnum<class "Interface.lvclass">)  [unwired: 7 in]
        n3634 = call-dynamic "Write Interface.vi"("error in (no error)"=w8453, "Interface.lvclass"=w8454, "Channel in"=w8460) -> ("error out"=w8459:errorcluster, "Channel out"=w8458:refnum<class "Channel.lvclass">)  [unwired: 7 in]
        n3635 = call-dynamic "Write Channel.vi"("error in (no error)"=w8459, "Channel.lvclass"=w8458, "Acquisition in"=w8457) -> ("error out"=w8463:errorcluster, "Acquisition out"=w8465:refnum<class "Acquisition.lvclass">)  [unwired: 7 in]
        n3636 = call-dynamic "Write AcquisitionC.vi"("error in (no error)"=w8463, "Acquisition.lvclass"=w8465, "S4ACS_GUI in"=w8464) -> ("error out"=w8449:errorcluster, "S4ACS_GUI out"=w8448:refnum<class "S4GUI.lvclass">)  [unwired: 7 in]
      }
      event "Exptime ch4": Value Change {
        n3637 = event-data() -> ("NewVal"=w8472:dbl)  [unwired: 1 in]
        n3638 = call-dynamic "Read AcquisitionD.vi"("error in (no error)"=w8471, "S4ACS_GUI in"=w8470) -> ("error out"=w8486:errorcluster, "Acquisition.lvclass"=w8487:refnum<class "Acquisition.lvclass">, "S4ACS_GUI out"=w8484:refnum<class "S4GUI.lvclass">)  [unwired: 7 in]
